vi "graph_error_response.vi"(8 "error in (no error)":errorcluster, 11 "Error Response":string="{\n   \"error\":{\n      \"code\":\"10002\",\n      \"message\":\"The service is currently unavailable. Please try again later.\",\n      \"innerError\": {\n        \"requestId\": \"request-id\",\n        \"date\": \"date-time\"\n      }\n   }\n}") -> (0 "error out":errorcluster, 3 "data":T1={"error"={"innerError"={"date"="date-time", "requestId"="request-id"}, "message"="The service is currently unavailable. Please try again later.", "code"="10002"}})   [LabVIEW 2016]
uses:
  <vilib>/addons/_JKI.lib/Serialization/JSON/JKI JSON Serialization.lvlib
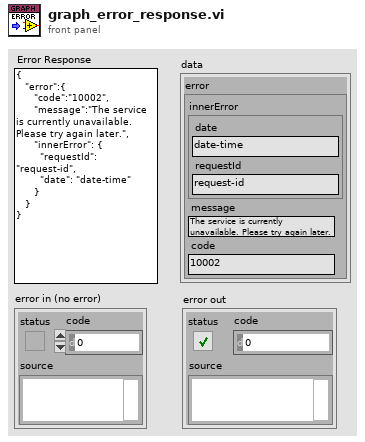
[diagram p1: front panel]
types:
  T1 = cluster{"error":cluster{"innerError":cluster{"date":string, "requestId":string}, "message":string, "code":string}}
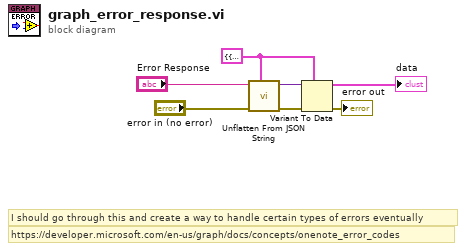
[diagram p0: block diagram]
diagram:
  w5 = T1 {"error"={"innerError"={"date"="", "requestId"=""}, "message"="", "code"=""}}
  # "I should go through this and create a way to handle certain types of errors eventually"
  # "https://developer.microsoft.com/en-us/graph/docs/concepts/onenote_error_codes"
  n1 = call <vilib>:"Unflatten From JSON String.vi"("Type and Defaults"=w5, "error in (no error)"="error in (no error)", "JSON String"="Error Response") -> ("error out"=w1:errorcluster, "Variant"=w6:variant)  [unwired: 7 in]
  n2 = Variant To Data(error in=w1, type=w5, Variant=w6) -> (data=→"data":T1, error out=→"error out":errorcluster)
